vi "LaserLineDetection_Intensity_distance.vi"(10 "Camera Parameters":T1, 11 "Pixel":dbl) -> (3 "Distance (D)":dbl)   [LabVIEW 2013]
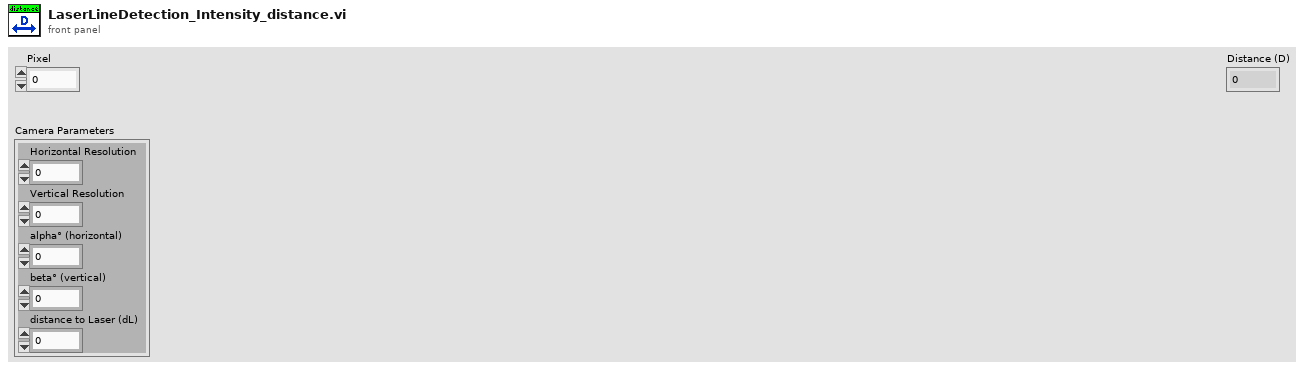
[diagram p1: front panel]
types:
  T1 = cluster{"Horizontal Resolution":dbl, "Vertical Resolution":dbl, "alpha° (horizontal)":dbl, "beta° (vertical)":dbl, "distance to Laser (dL)":dbl}
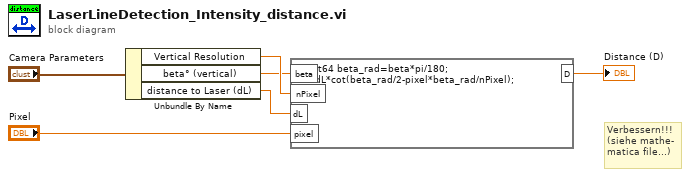
[diagram p0: block diagram]
diagram:
  # "Verbessern!!!\n(siehe mathe-\nmatica file...)"
  n1 = Unbundle By Name("Camera Parameters") -> ("Vertical Resolution"=w6:dbl, "beta° (vertical)"=w4:dbl, "distance to Laser (dL)"=w5:dbl)
  n2 = formula code="float64 beta_rad=beta*pi/180;\nD=dL*cot(beta_rad/2-pixel*beta_rad/nPixel);"("pixel"="Pixel", "beta"=w4, "nPixel"=w6, "dL"=w5) -> ("D"=→"Distance (D)":dbl)
